vi "GetErrorCreationType.vi"(8 "ErrorIn":errorcluster) -> (0 "ErrorOut":errorcluster, 1 "ErrorCreationType":refnum<class "ErrorCreationExecution.lvclass">)   [LabVIEW 2021, in "ErrorCreationExecution.lvclass"]
uses:
  ErrorCreationExecution.lvclass
  ErrorCreationType.vi
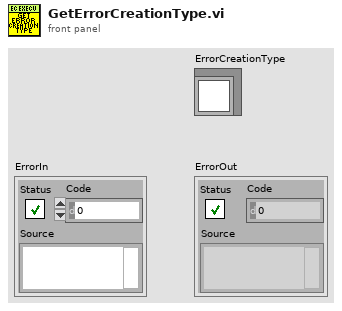
[diagram p1: front panel]
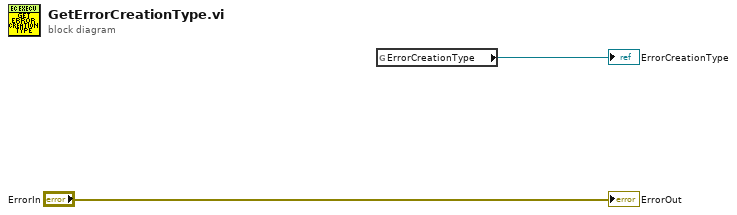
[diagram p0: block diagram]
diagram:
  n1 = global read "ErrorCreationType.vi" "ErrorCreationType"() -> (→"ErrorCreationType":refnum<class "ErrorCreationExecution.lvclass">)
  "ErrorOut" <- "ErrorIn"
